vi "Build Error File Path and Create Folder.vi"(7 "File Name":string, 8 "error in (no error)":errorcluster, 11 "Base Path":path) -> (0 "error out":errorcluster, 2 "Result File path":path, 3 "Result Folder path":path)   [LabVIEW 2022 SP3]
doc: "Copyright © 2011, Unilogic Technologies.\nAll rights reserved."
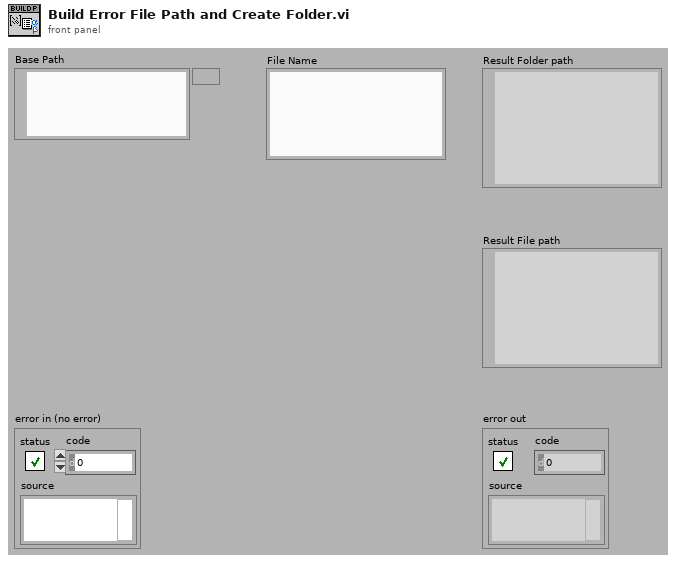
[diagram p1: front panel]
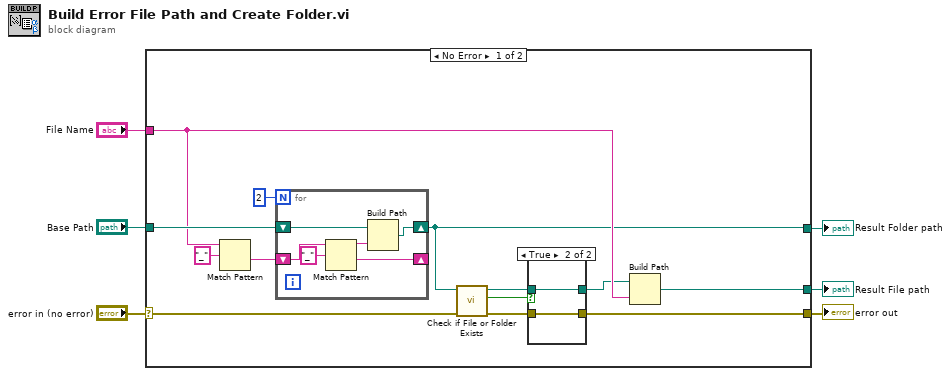
[diagram p0: block diagram]
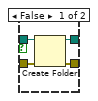
[diagram p2: hidden frame]
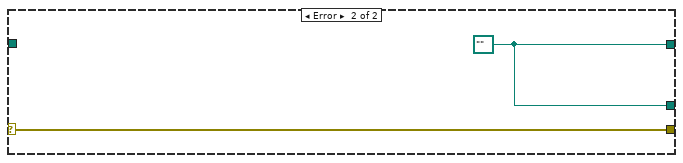
[diagram p3: hidden frame]
diagram:
  n1 = case shown="No Error" "error in (no error)" {
    selector: "error in (no error)" -> [w11 w33]
    tunnel: [w14 w33] -> w5
    tunnel: [w10 w32] -> w4
    tunnel: [w13 w32] -> w3
    tunnel: "File Name" -> [w16 _]
    tunnel: "Base Path" -> [w18 _]
    frame No Error {
      n2 = Match Pattern(string=w16, regular expression="_" ("search string/char (-)")) -> (after substring=w15:string)  [unwired: 1 in, 3 out]
      n3 = for {
        N: 2 -> [_]
        shift-right: [w26] -> _
        shift-left: w15 -> [w30]
        shift-right: [w27] -> w10
        shift-left: w18 -> [w29]
        n4 = Match Pattern(string=w30, regular expression="_" ("search string/char (-)")) -> (before substring=w28:string, after substring=w26:string)  [unwired: 1 in, 2 out]
        n5 = Build Path(base path=w29, name or relative path=w28) -> (appended path=w27:path)
      }
      n6 = call <vilib>:"Check if File or Folder Exists.vi"("error in (no error)"=w11, "path"=w10) -> ("error out"=w8:errorcluster, "file or folder exists?"=w7:bool, "dup path"=w9:path)  [unwired: 7 in]
      n7 = case shown="True" w7 {
        tunnel: [w23 w24] -> w14
        tunnel: [w22 w25] -> w12
        tunnel: w9 -> [w21 w25]
        tunnel: w8 -> [w20 w24]
        frame False {
          n8 = Create Folder(path (use dialog)=w21, error in=w20) -> (created path=w22:path, error out=w23:errorcluster)  [unwired: 1 in, 1 out]
        }
        frame True {
        }
      }
      n9 = Build Path(base path=w12, name or relative path=w16) -> (appended path=w13:path)
    }
    frame Error {
      w32 = path "" ("appended path")
    }
  }
  "error out" <- w5
  "Result Folder path" <- w4
  "Result File path" <- w3
